vi "Spawn.vi"(6 "Transport":refnum<class "Transport.lvclass">, 7 "Actor in":refnum<class "Actor.lvclass">, 9 "UID":string, 10 "Actor":refnum<class "Actor.lvclass">) -> (0 "Error out":errorcluster, 5 "Actor out":refnum<class "Actor.lvclass">)   [LabVIEW 2025, in "jettl.lvlib"]
uses:
  jettl.lvlib
  Actor/Actor.lvclass
  Transport/Transport/Transport.lvclass
  Error/Error.lvlib
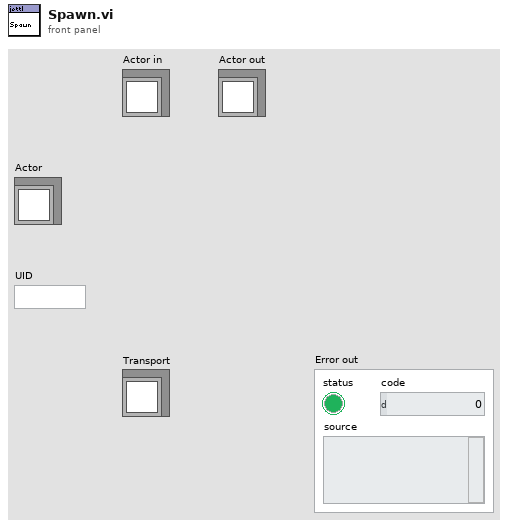
[diagram p1: front panel]
types:
  T1 = typedef "jettl.lvlib/Child UIDs.ctl" = set{string}
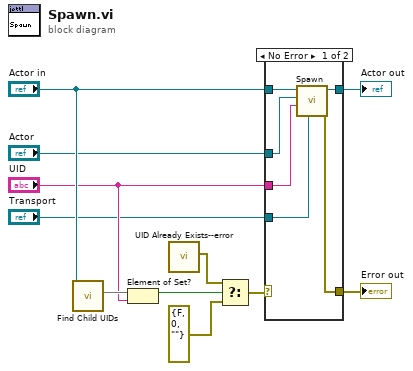
[diagram p0: block diagram]
diagram:
  n1 = call-dynamic "Find Child UIDs.vi"("Actor in"="Actor in") -> ("Child UIDs"=w9:T1)  [unwired: 10 in]
  n2 = Element of Set?(10:"UID", 11:w9) -> (3:w5:bool)
  n3 = call "UID Already Exists--error.vi"() -> ("Error"=w6:errorcluster)  [unwired: 11 in]
  n4 = Select(t=w6, s=w5, f=errorcluster {"status"=FALSE, "code"=0, "source"=""}) -> (s? t:f=w3:errorcluster)
  n5 = case shown="No Error" w3 {
    selector: w3 -> [_ w18]
    tunnel: "UID" -> [w13 _]
    tunnel: "Actor in" -> [w15 w19]
    tunnel: [w17 w18] -> w11
    tunnel: [w16 w19] -> w10
    tunnel: "Actor" -> [w14 _]
    tunnel: "Transport" -> [w12 _]
    frame No Error {
      n6 = call-dynamic "Spawn.vi"("Transport"=w12, "UID"=w13, "Actor"=w14, "Actor in"=w15) -> ("Error out"=w17:errorcluster, "Actor out"=w16:refnum<class "Actor.lvclass">)  [unwired: 6 in]
    }
    frame Error {
    }
  }
  "Error out" <- w11
  "Actor out" <- w10
